vi "ScanDelay_FTIR_GetSpectrum_Aligning_ProducerConsumer.vi"(0 "Cancel? External":refnum<vi>, 1 "% averaged (external)":refnum<vi>, 2 "Binned interferogram (external)":refnum<vi>, 3 "Python refnum in":refnum<k35>, 5 "Refresh alignment":bool=TRUE, 7 "Acquisition cycle (external)":refnum<vi>, 9 "Delay calibration\n          factor":dbl=2.403, 10 "Python error in":errorcluster, 11 "Subtract\ndelay (ps)":dbl, 12 "Acquisitions per interferogram":i32=50, 13 "Time per\nacquisition (s)":dbl=0.2, 14 "Sampling rate":dbl=250000.0, 15 "Extract envelope":bool=TRUE) -> (4 "Output spectrum":dbl[][](array[numeric]), 6 "Python error out":errorcluster)   [LabVIEW 2021]
uses:
  Control_GetSpectrum_Aligning.ctl
  <vilib>/DAQmx/read.llb/DAQmx Read (Analog 2D DBL NChan NSamp).vi
  <vilib>/DAQmx/miscellaneous.llb/DAQmx Fill In Error Info.vi
panel:
  out "DAQmx error":errorcluster
  out "Time per\nloop (ms)":dbl
  in  "Save interferograms\n(interferograms.txt)":bool
  in  "Alignment order":i32=2
  out "Own python session":bool
  out "Refnum errors":errorcluster
  out "Spectrum (amplitude)":cluster{dbl[], dbl[]}[](graph)
  out "Spectrum (phase)":cluster{dbl[], dbl[]}(graph)
  out "Interferogram (aligned)":cluster{dbl, dbl}[](graph)
  out "% averaged":dbl=100.0
  out "Acquisition cycle":dbl[][](graph)
  in  "Halt acquisition":bool
  out "Python module path":path=path "C:/Users/mnopl/Desktop/Software/LabVIEW/ScanDelay/scandelay.py"
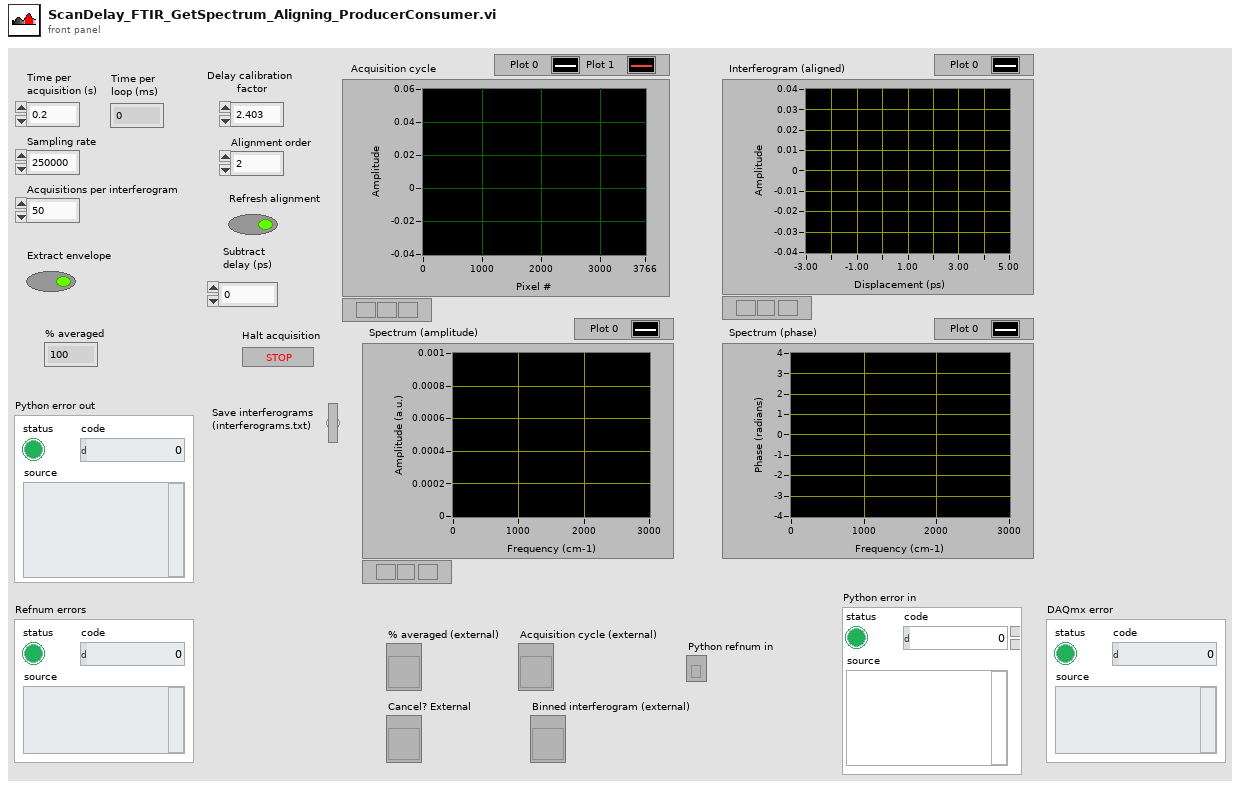
[diagram p1: front panel]
types:
  T1 = typedef "Control_GetSpectrum_Aligning.ctl" = enum16{"Acquire Interferograms", "Prepare DAQ task", "Align Interferograms", "Compute Spectrum", "Done"}
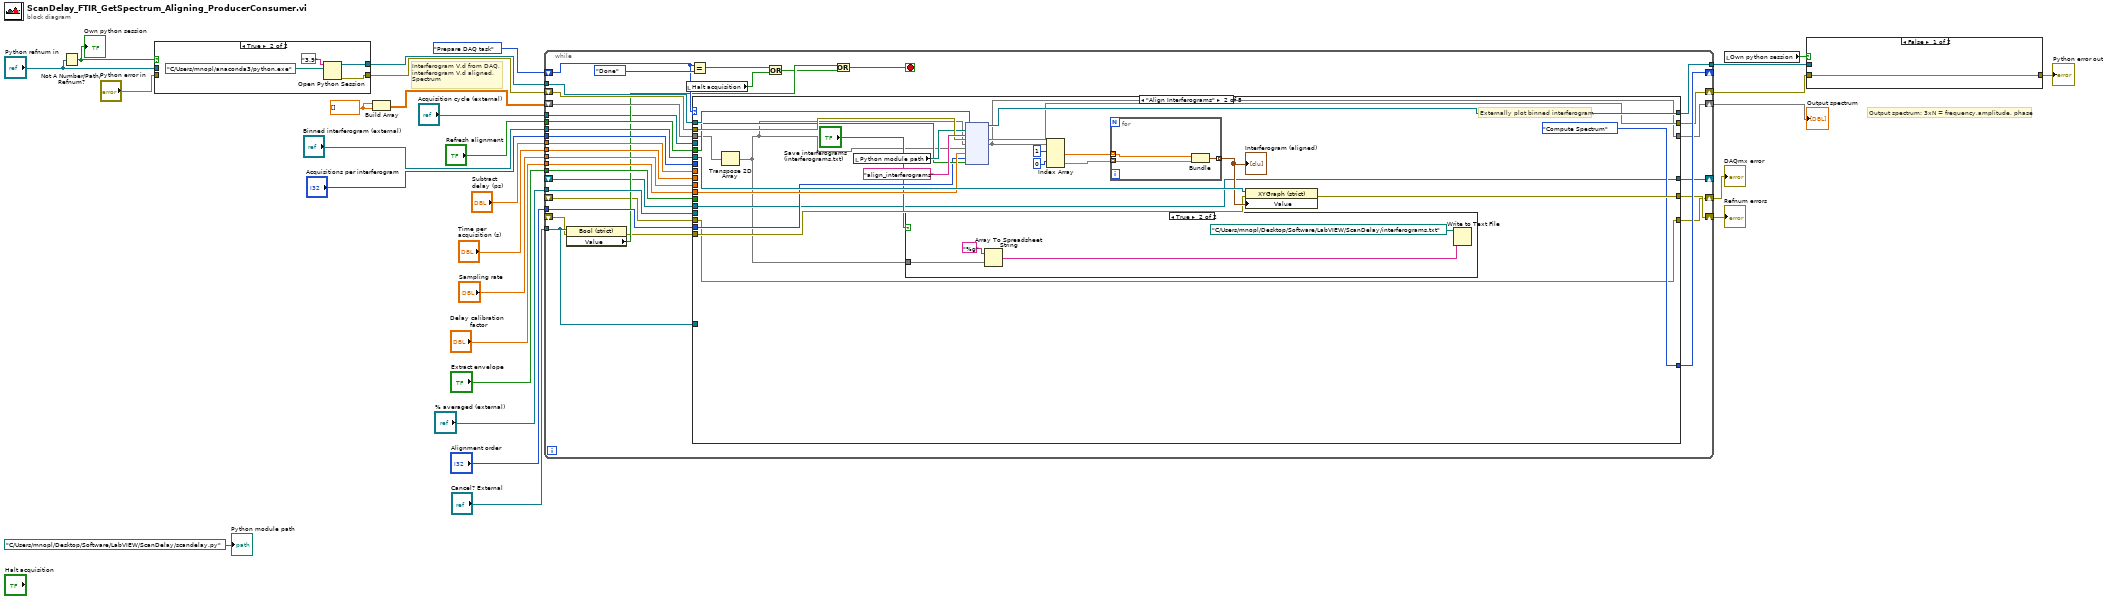
[diagram p0: block diagram]
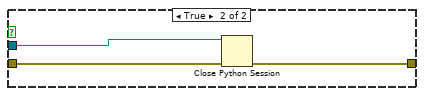
[diagram p2: hidden frame]
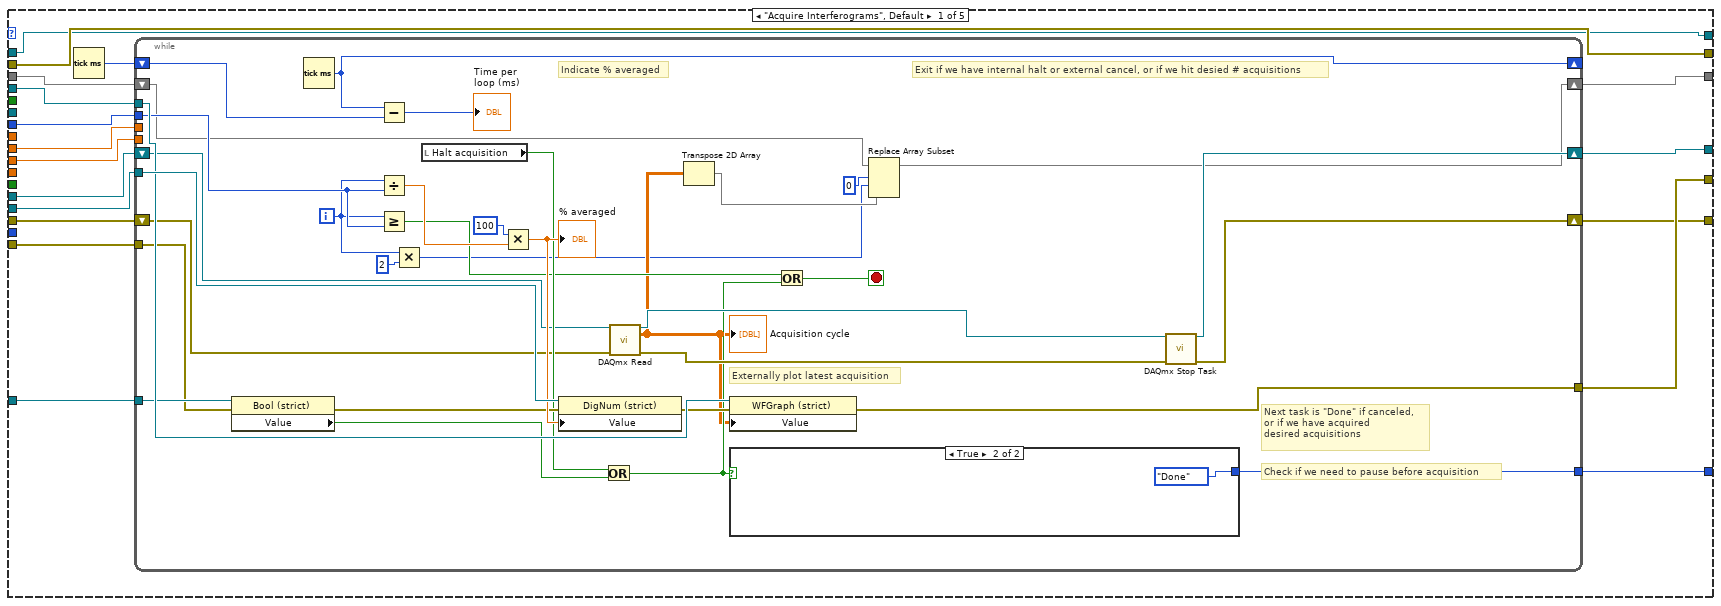
[diagram p4: hidden frame]
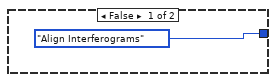
[diagram p5: hidden frame]
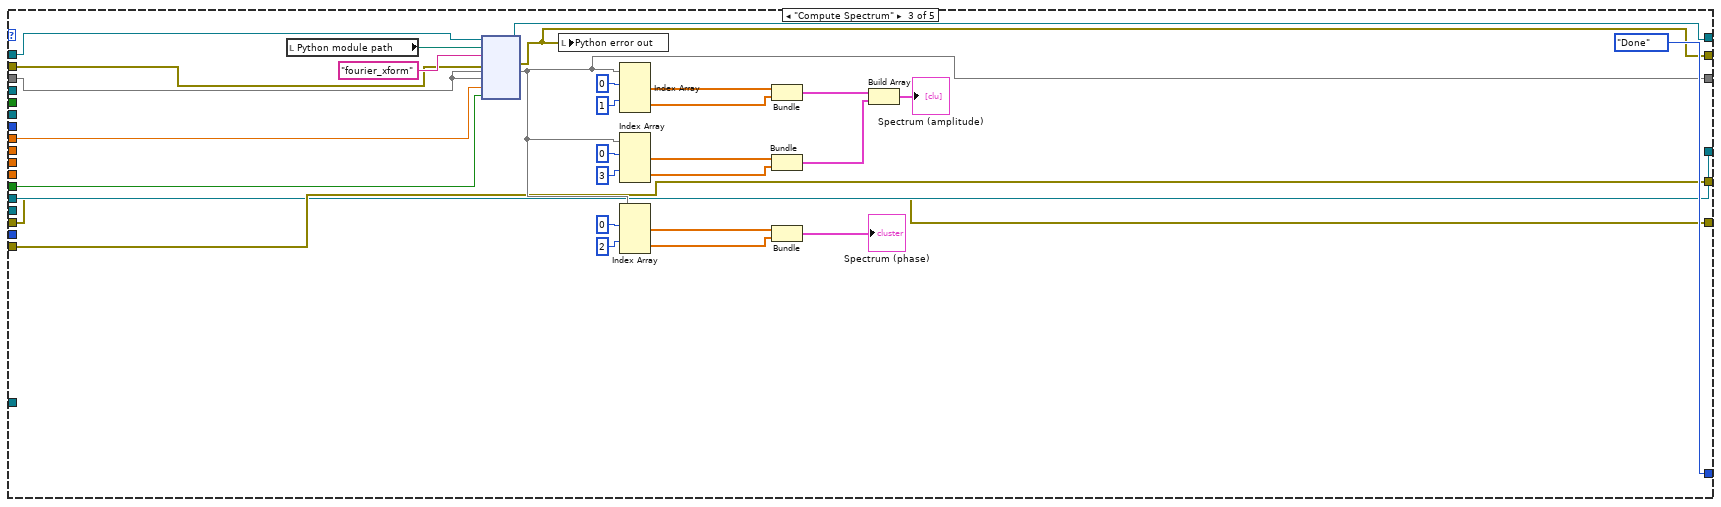
[diagram p7: hidden frame]
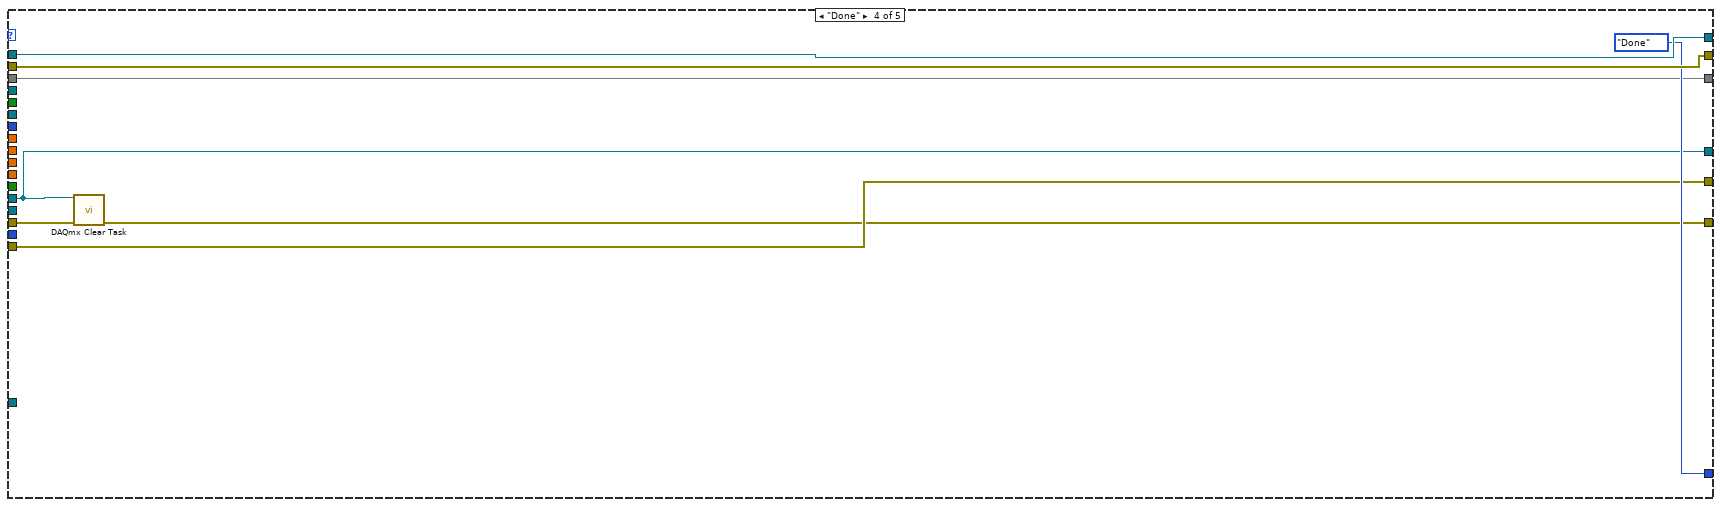
[diagram p8: hidden frame]
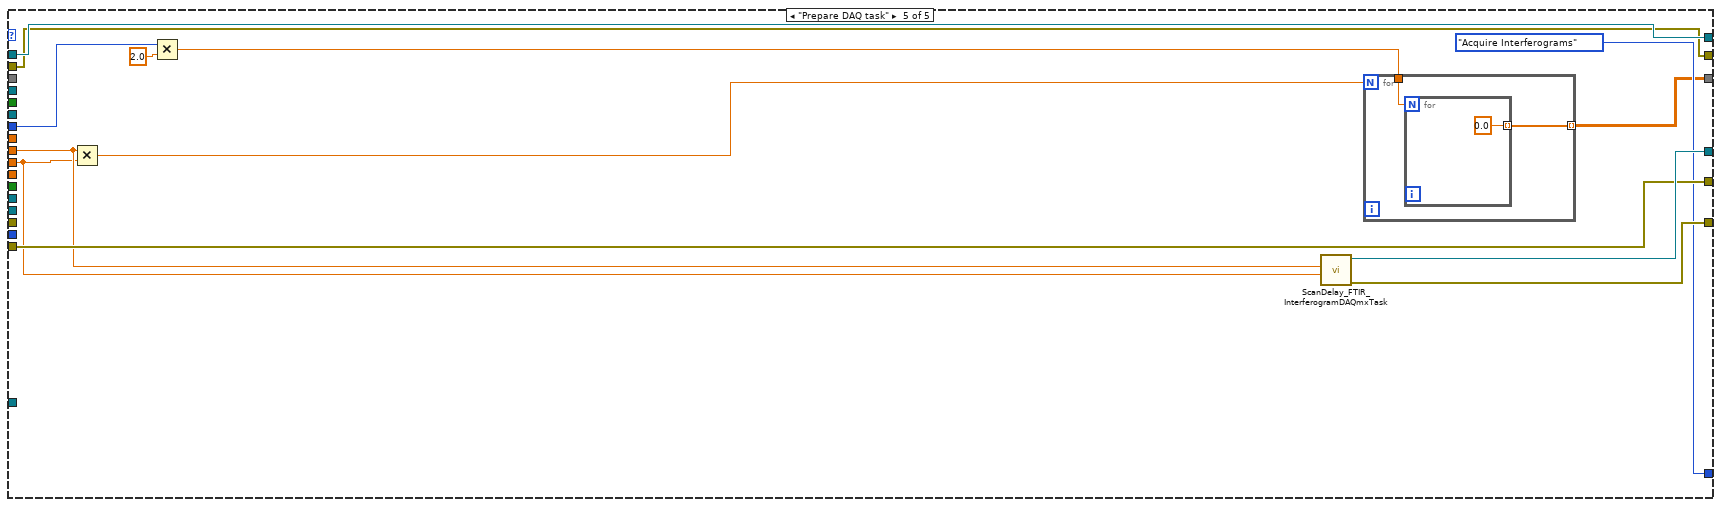
[diagram p9: hidden frame]
diagram:
  w17 = dbl[] []
  # "Output spectrum: 3xN = frequency,amplitude, phase"
  # "Interferogram V,d from DAQ,\ninterferogram V,d aligned,\nSpectrum"
  n1 = Not A Number/Path/Refnum?(number/path/refnum="Python refnum in") -> (NaN/Path/Refnum?=w7:bool)
  "Own python session" <- w7
  n2 = case shown="True" w7 {
    tunnel: [w30 w32] -> w11
    tunnel: [w29 w31] -> w10
    tunnel: "Python refnum in" -> [w30 _]
    tunnel: "Python error in" -> [w29 _]
    frame False {
    }
    frame True {
      n3 = Open Python Session(python version="3.9", python path=path "C:/Users/mnopl/anaconda3/python.exe") -> (session out=w32:refnum<k35>, error out=w31:errorcluster)  [unwired: 1 in]
    }
  }
  n4 = Build Array(w17, w17) -> (w4:dbl[][])
  n5 = while {
    shift-right: [w49] -> w16
    shift-left: w4 -> [w67]
    tunnel: w11 -> [w66]
    tunnel: "Acquisition cycle (external)" -> [w39]
    tunnel: "Sampling rate" -> [w64]
    tunnel: "Time per\nacquisition (s)" -> [w63]
    tunnel: "Delay calibration\n          factor" -> [w62]
    tunnel: "% averaged (external)" -> [w61]
    tunnel: "Cancel? External" -> [w42]
    tunnel: "Acquisitions per interferogram" -> [w60]
    shift-right: [w59] -> _
    shift-left: Control_GetSpectrum_Aligning."Prepare DAQ task" -> [w50]
    tunnel: "Subtract\ndelay (ps)" -> [w58]
    tunnel: [w55] -> w18
    shift-right: [w54] -> w15
    shift-left: w10 -> [w65]
    tunnel: "Extract envelope" -> [w53]
    shift-right: [w52] -> w13
    shift-left: _ -> [w40]
    tunnel: "Binned interferogram (external)" -> [w51]
    tunnel: "Refresh alignment" -> [w48]
    tunnel: "Alignment order" -> [w47]
    shift-right: [w37] -> w1
    shift-left: _ -> [w35]
    shift-right: [w38] -> _
    shift-left: _ -> [w36]
    stop <- w44 stop-if-true
    n6 = property on="Property Node" class="Bool (strict)"(reference=w42, error in=w40) -> (error out=w41:errorcluster, "Value"=w46:bool)  [unwired: 1 out]
    n7 = local read "Halt acquisition"() -> (w43:bool)
    n8 = Equal?(x=w50, y=Control_GetSpectrum_Aligning."Done") -> (x = y?=w56:bool)
    n9 = case shown="\"Align Interferograms\"" w50 {
      tunnel: w67 -> [w68 w123 w181 w187 _]
      tunnel: w66 -> [w70 w144 w180 w189 w199]
      tunnel: w65 -> [w80 w143 w177 w190 w198]
      tunnel: w39 -> [w85 _ _ _ _]
      tunnel: w64 -> [w84 _ _ _ w193]
      tunnel: w63 -> [w83 _ _ _ w197]
      tunnel: w62 -> [_ w131 _ _ _]
      tunnel: w61 -> [w82 _ _ _ _]
      tunnel: w42 -> [w81 _ _ _ _]
      tunnel: w60 -> [w77 _ _ _ w194]
      tunnel: [w70 w142 w179 w189 w199] -> w55
      tunnel: [w75 Control_GetSpectrum_Aligning."Compute Spectrum" Control_GetSpectrum_Aligning."Done" Control_GetSpectrum_Aligning."Done" Control_GetSpectrum_Aligning."Acquire Interferograms"] -> w59
      tunnel: w58 -> [_ _ w176 _ _]
      tunnel: [w80 w138 w157 w190 w198] -> w54
      tunnel: w53 -> [_ _ w166 _ _]
      tunnel: [w79 w136 w155 w186 w201] -> w52
      tunnel: w51 -> [_ w137 _ _ _]
      tunnel: [w78 w130 w156 w187 w196] -> w49
      tunnel: w48 -> [_ w129 _ _ _]
      tunnel: w47 -> [_ w128 _ _ _]
      tunnel: w41 -> [w76 w127 w155 w186 w201]
      tunnel: [w72 w125 w154 w185 w203] -> w38
      tunnel: [w71 w124 w153 w183 w202] -> w37
      tunnel: w36 -> [w74 w125 w154 w185 _]
      tunnel: w35 -> [w73 w124 w153 w184 _]
      frame "Acquire Interferograms", Default {
        n10 = Tick Count (ms)() -> (millisecond timer value=w69:u32)
        n11 = while {
          tunnel: w85 -> [w115]
          tunnel: w84 -> [_]
          tunnel: w83 -> [_]
          tunnel: w82 -> [w117]
          tunnel: w81 -> [w112]
          tunnel: [w113] -> w79
          shift-right: [w93] -> w78
          shift-left: w68 -> [w92]
          tunnel: w77 -> [w105]
          tunnel: w76 -> [w111]
          tunnel: [w108] -> w75
          shift-right: [w99] -> w72
          shift-left: w74 -> [w104]
          shift-right: [w100] -> w71
          shift-left: w73 -> [w103]
          shift-right: [w98] -> _
          shift-left: w69 -> [w97]
          i -> [w95]
          stop <- w109 stop-if-true
          # "Next task is \"Done\" if canceled,\nor if we have acquired \ndesired acquisitions"
          # "Exit if we have internal halt or external cancel, or if we hit desied # acquisitions"
          # "Externally plot latest acquisition"
          # "Indicate % averaged"
          # "Check if we need to pause before acquisition"
          n12 = property on="Property Node" class="Bool (strict)"(reference=w112, error in=w111) -> (error out=w110:errorcluster, "Value"=w107:bool)  [unwired: 1 out]
          n13 = Tick Count (ms)() -> (millisecond timer value=w98:u32)
          n14 = Subtract(x=w98, y=w97) -> (x-y=→"Time per\nloop (ms)":u32)
          n15 = Divide(x=w95, y=w105) -> (x/y=w119:dbl)
          n16 = Greater Or Equal?(x=w95, y=w105) -> (x >= y?=w90:bool)
          n17 = Multiply(x=w95, y=2) -> (x*y=w86:i32)
          n18 = local read "Halt acquisition"() -> (w106:bool)
          n19 = Multiply(x=100, y=w119) -> (x*y=w116:dbl)
          "% averaged" <- w116
          n20 = property on="Property Node" class="DigNum (strict)"(reference=w117, error in=w110, "Value"=w116) -> (error out=w114:errorcluster)  [unwired: 1 out]
          n21 = Or(x=w106, y=w107) -> (x .or. y?=w91:bool)
          n22 = call-poly <vilib>:"DAQmx Read.vi"("task/channels in"=w104, "error in"=w103) -> ("task out"=w102:refnum<k21>, "data"=w88:dbl[][], "error out"=w101:errorcluster)  [unwired: 11 in]
          "Acquisition cycle" <- w88
          n23 = Transpose 2D Array(2D array=w88) -> (transposed array=w89:dbl[][])
          n24 = property on="Property Node" class="WFGraph (strict)"(reference=w115, error in=w114, "Value"=w88) -> (error out=w113:errorcluster)  [unwired: 1 out]
          n25 = case shown="True" w91 {
            tunnel: [Control_GetSpectrum_Aligning."Align Interferograms" Control_GetSpectrum_Aligning."Done"] -> w108
            frame False {
            }
            frame True {
            }
          }
          n26 = Or(x=w90, y=w91) -> (x .or. y?=w109:bool)
          n27 = Replace Array Subset(array=w92, new element=w89, index (row)=0, index (col)=w86) -> (w93:dbl[][])
          n28 = call <vilib>:"DAQmx Stop Task.vi"("task/channels in"=w102, "error in"=w101) -> ("task out"=w99:refnum<k21>, "error out"=w100:errorcluster)  [unwired: 12 in]
        }
      }
      frame "Align Interferograms" {
        # "Externally plot binned interferogram"
        n29 = Transpose 2D Array(2D array=w123) -> (transposed array=w122:dbl[][])
        n30 = local read "Python module path"() -> (w141:path)
        n31 = case shown="True" "Save interferograms\n(interferograms.txt)" {
          tunnel: w122 -> [_ w147]
          frame False {
          }
          frame True {
            n32 = Array To Spreadsheet String(array=w147, 3:"%g") -> (spreadsheet string=w149:string)  [unwired: 1 in]
            n33 = Write to Text File(file (use dialog)=path "C:/Users/mnopl/Desktop/Software/LabVIEW/ScanDelay/interferograms.txt", text=w149) -> ()  [unwired: 2 in, 3 out]
          }
        }
        n34 = node(w144, w141, "align_interferograms", w143, w122, w122, w131, w128, w129) -> (w142:refnum<k35>, w138:errorcluster, w130:dbl[][])  [unwired: 4 in, 2 out]
        n35 = Index Array(array=w130, index (row) #1=1, index (row) #2=0) -> (element #1=w134:dbl[], element #2=w135:dbl[])  [unwired: 2 in]
        n36 = for {
          tunnel: w135 -> [w151] mode=indexing
          tunnel: w134 -> [w152] mode=indexing
          tunnel: [w150] -> w133 mode=indexing
          n37 = Bundle(w152, w151) -> (w150:cluster{dbl, dbl})  [unwired: 1 in]
        }
        "Interferogram (aligned)" <- w133
        n38 = property on="Property Node" class="XYGraph (strict)"(reference=w137, error in=w127, "Value"=w133) -> (error out=w136:errorcluster)  [unwired: 1 out]
      }
      frame "Compute Spectrum" {
        n39 = local read "Python module path"() -> (w178:path)
        n40 = node(w180, w178, "fourier_xform", w177, w181, w181, w176, w166) -> (w179:refnum<k35>, w157:errorcluster, w156:dbl[][])  [unwired: 3 in, 2 out]
        n41 = local write "Python error out"(w157) -> ()
        n42 = Index Array(array=w156, index (row) #1=0, index (row) #2=1) -> (element #1=w172:dbl[], element #2=w171:dbl[])  [unwired: 2 in]
        n43 = Index Array(array=w156, index (row) #1=0, index (row) #2=3) -> (element #1=w167:dbl[], element #2=w168:dbl[])  [unwired: 2 in]
        n44 = Index Array(array=w156, index (row) #1=0, index (row) #2=2) -> (element #1=w162:dbl[], element #2=w163:dbl[])  [unwired: 2 in]
        n45 = Bundle(w172, w171) -> (w160:cluster{dbl[], dbl[]})  [unwired: 1 in]
        n46 = Bundle(w167, w168) -> (w159:cluster{dbl[], dbl[]})  [unwired: 1 in]
        n47 = Bundle(w162, w163) -> (→"Spectrum (phase)":cluster{dbl[], dbl[]})  [unwired: 1 in]
        n48 = Build Array(w160, w159) -> (→"Spectrum (amplitude)":cluster{dbl[], dbl[]}[])
      }
      frame "Done" {
        n49 = call <vilib>:"DAQmx Clear Task.vi"("task in"=w185, "error in"=w184) -> ("error out"=w183:errorcluster)  [unwired: 13 in]
      }
      frame "Prepare DAQ task" {
        n50 = Multiply(x=w197, y=w193) -> (x*y=w192:dbl)
        n51 = Multiply(x=w194, y=2.0) -> (x*y=w191:dbl)
        n52 = call "ScanDelay_FTIR_InterferogramDAQmxTask.vi"("Sampling rate"=w193, "Time per acquisiton (s)"=w197) -> ("error out"=w202:errorcluster, "Refnum out"=w203:refnum<k21>)  [unwired: 8 in]
        n53 = for {
          N: w192 -> [_]
          tunnel: [w205] -> w196 mode=indexing
          tunnel: w191 -> [w204]
          n54 = for {
            N: w204 -> [_]
            tunnel: [0.0] -> w205 mode=indexing
          }
        }
      }
    }
    n55 = Or(x=w56, y=w43) -> (x .or. y?=w45:bool)
    n56 = Or(x=w46, y=w45) -> (x .or. y?=w44:bool)
  }
  "Output spectrum" <- w16
  "Refnum errors" <- w13
  "DAQmx error" <- w1
  n57 = local read "Own python session"() -> (w6:bool)
  n58 = case shown="False" w6 {
    tunnel: [w207 w210] -> w19
    tunnel: w18 -> [_ w209]
    tunnel: w15 -> [w207 w208]
    frame False {
    }
    frame True {
      n59 = Close Python Session(session in=w209, error in=w208) -> (11:w210:errorcluster)
    }
  }
  "Python error out" <- w19
  "Python module path" <- path "C:/Users/mnopl/Desktop/Software/LabVIEW/ScanDelay/scandelay.py"
